vi "OverlayRectangleCenterSize.vi"(4 "Color":u32(colorbox)=16711680, 6 "Drawing Mode (Frame)":T2, 7 "GroupName":string, 8 "error in":errorcluster, 9 "Size":T1, 10 "Center-Point":T1, 11 "Image Reference In":T3) -> (0 "error out":errorcluster, 3 "Image Reference Out":T3)   [LabVIEW 2024, in "OpenLvVision_Overlays.lvlib"]
doc: "Overlays an rectangle on top of an image.\nDraws the rectangle arround a center point."
uses:
  OpenLvVision_Overlays.lvlib
  <vilib>/OpenLvVision/OpenLvVision_Image/Management/TypeDef/OLV Image.ctl
  TypeDefs/DrawingMode.ctl
  TypeDefs/PointI32.ctl
  <vilib>/OpenLvVision/OpenLvVision_Image/Management/OLV Management.lvlib
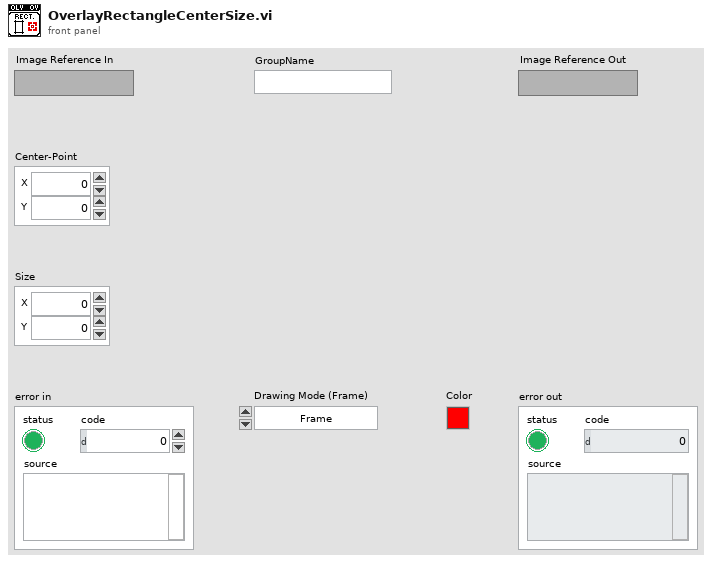
[diagram p1: front panel]
types:
  T1 = typedef "OpenLvVision_Overlays.lvlib/PointI32.ctl" = cluster{"X":i32, "Y":i32}
  T2 = typedef "OpenLvVision_Overlays.lvlib/DrawingMode.ctl" = enum16{"Frame", "Fill"}
  T3 = typedef "OLV OpenLvVision_Image.lvlib/OLV Management.lvlib/OLV Image.ctl" = refnum<image>
  T4 = typedef "OLV OpenLvVision_Image.lvlib/OLV DataAccess.lvlib/OLV RectangleI32.ctl" = cluster{"Left":i32, "Top":i32, "Right":i32, "Bottom":i32}
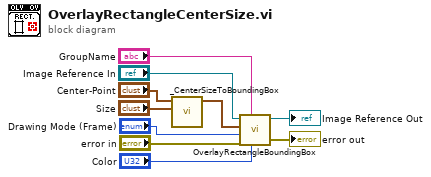
[diagram p0: block diagram]
diagram:
  n1 = call "_CenterSizeToBoundingBox.vi"("Size"="Size", "Center-Point"="Center-Point") -> ("Bounding Box"=w1:T4)  [unwired: 9 in]
  n2 = call "OverlayRectangleBoundingBox.vi"("Color"="Color", "GroupName"="GroupName", "error in"="error in", "Drawing Mode (Frame)"="Drawing Mode (Frame)", "Rectangle"=w1, "Image Reference In"="Image Reference In") -> ("error out"=→"error out":errorcluster, "Image Reference Out"=→"Image Reference Out":T3)  [unwired: 4 in]
